vi "Set State.vi"(8 "Error In":errorcluster, 10 "Data":variant, 11 "States":T1=enum."SCAN") -> (0 "Error Out":errorcluster)   [LabVIEW 2014]
uses:
  Controls/StateControl.ctl
  Controls/State Typedef.ctl
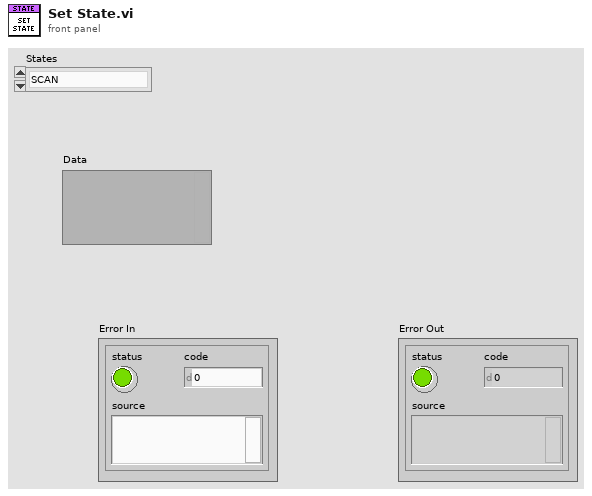
[diagram p1: front panel]
types:
  T1 = typedef "StateControl.ctl" = enum16{"WAIT FOR EVENT", "GET HEALTH", "SCAN", "RESET", "EXIT"}
  T2 = typedef "State Typedef.ctl" = cluster{"State":T1, "Data":variant}
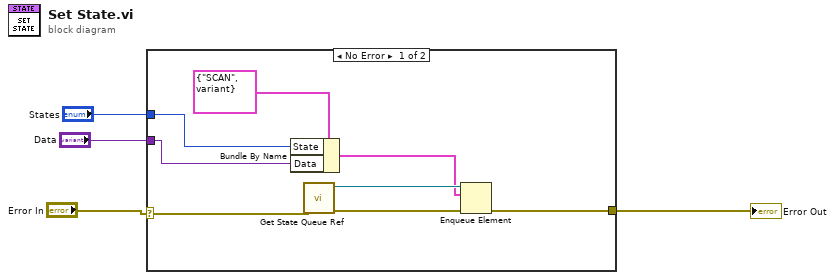
[diagram p0: block diagram]
diagram:
  n1 = case shown="No Error" "Error In" {
    selector: "Error In" -> [w9 w13]
    tunnel: "Data" -> [w10 _]
    tunnel: "States" -> [w11 _]
    tunnel: [w5 w13] -> w1
    frame No Error {
      n2 = Bundle By Name(cluster=T2 {"State"=enum."SCAN", "Data"=variant} ("State Control"), "State"=w11, "Data"=w10) -> (w6:T2)
      n3 = call "Get State Queue Ref.vi"("error in (no error)"=w9) -> ("error out"=w8:errorcluster, "queue out"=w7:refnum<queue>)  [unwired: 9 in]
      n4 = Enqueue Element(queue=w7, element=w6, error in (no error)=w8) -> (error out=w5:errorcluster)  [unwired: 1 in, 2 out]
    }
    frame Error {
    }
  }
  "Error Out" <- w1
